vi "Read Inputs.vi"(8 "error in (no error)":errorcluster, 11 "PLBB in":refnum<class "Test Device.lvclass">) -> (0 "error out":errorcluster, 2 "inputs":T1, 3 "PLBB out":refnum<class "Test Device.lvclass">)   [LabVIEW 2015, in "Test Device.lvclass"]
uses:
  Test Device.lvclass
  <vilib>/plasmapper/PL Modbus Client/PL Modbus Client.lvclass
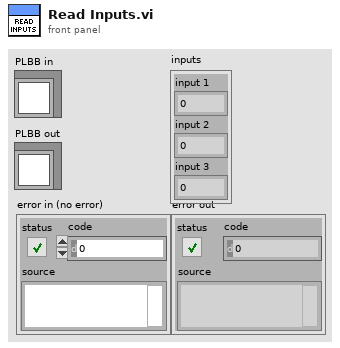
[diagram p1: front panel]
types:
  T1 = cluster{"input 1":u16, "input 2":u16, "input 3":u16}
  T2 = cluster{"values[0]":u16, "values[1]":u16, "values[2]":u16}
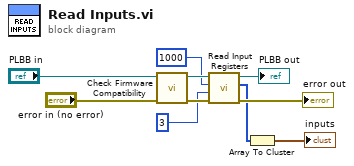
[diagram p0: block diagram]
diagram:
  n1 = call-dynamic "Check Firmware Compatibility.vi"("error in (no error)"="error in (no error)", "TD in"="PLBB in") -> ("error out"=w8:errorcluster, "TD out"=w7:refnum<class "Test Device.lvclass">)  [unwired: 8 in]
  n2 = call <vilib>:"Read Input Registers.vi"("error in (no error)"=w8, "number of input registers"=u16 3, "address"=u16 1000, "MODBUS in"=w7) -> ("error out"=→"error out":errorcluster, "values"=w2:u16[], "MODBUS out"=→"PLBB out":refnum<class "Test Device.lvclass">)  [unwired: 5 in]
  n3 = Array To Cluster(array=w2) -> (cluster=→"inputs":T2)
